vi "HK Channel Add Channel.vi"(8 "error in (no error)":errorcluster, 9 "HK Item.lvclass":refnum<class "HK Item.lvclass">, 11 "HK Channel in":refnum<class "HK Table.lvclass">) -> (0 "error out":errorcluster, 3 "HK Channel out":refnum<class "HK Table.lvclass">)   [LabVIEW 2019, in "HK Table.lvclass"]
uses:
  HK Table.lvclass
  HK Item/HK Item.lvclass
  HK Item/HK Item.lvclass/HK Item.ctl
  HK Table.lvclass/HK Table.ctl
  HK Item/HK Channel Read Name.vi
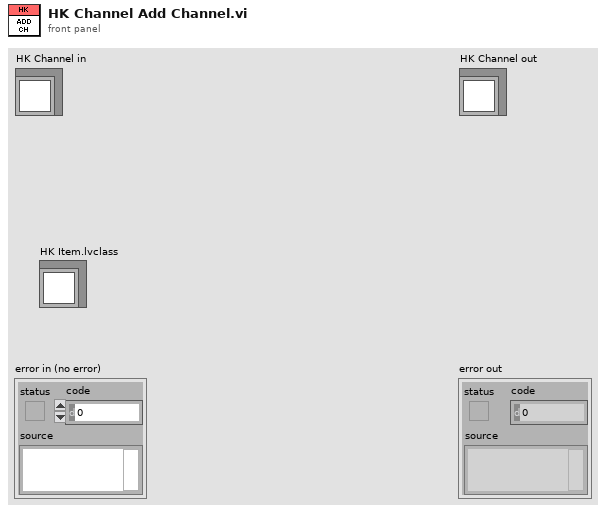
[diagram p1: front panel]
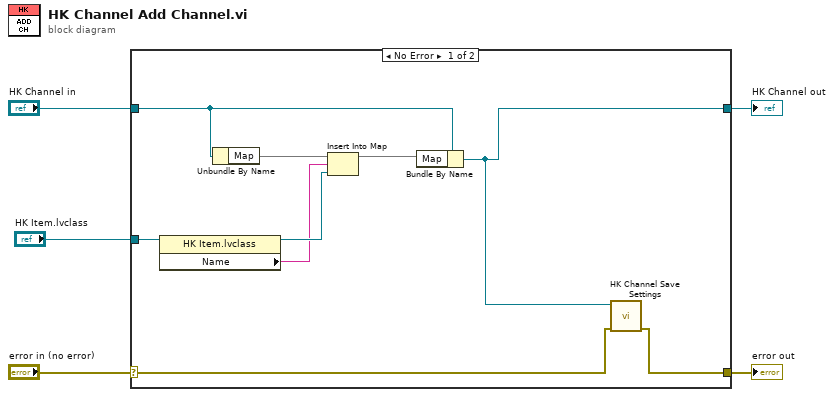
[diagram p0: block diagram]
diagram:
  n1 = case shown="No Error" "error in (no error)" {
    selector: "error in (no error)" -> [w10 w16]
    tunnel: [w9 w16] -> w4
    tunnel: [w11 w15] -> w2
    tunnel: "HK Channel in" -> [w12 w15]
    tunnel: "HK Item.lvclass" -> [w7 _]
    frame No Error {
      n2 = property class="HK Item.lvclass"(reference=w7) -> (reference out=w8:refnum<class "HK Item.lvclass">, "Name"=w6:string)  [unwired: 1 in, 1 out]
      n3 = Unbundle By Name(w12) -> ("Map"=w14:map{string, refnum<class "HK Item.lvclass">})
      n4 = Insert Into Map(map in=w14, key=w6, value=w8) -> (map out=w13:map{string, refnum<class "HK Item.lvclass">})  [unwired: 2 out]
      n5 = Bundle By Name(cluster=w12, "Map"=w13) -> (w11:refnum<class "HK Table.lvclass">)
      n6 = call-dynamic "HK Channel Save Settings.vi"("error in (no error)"=w10, "HK Channel in"=w11) -> ("error out"=w9:errorcluster)  [unwired: 7 in, 2 out]
    }
    frame Error {
    }
  }
  "error out" <- w4
  "HK Channel out" <- w2
